vi "Deploy.vi"(8 "error in (no error)":errorcluster, 11 "SDIST in":refnum<class "NI_AB_API_DSDIST.lvclass">) -> (0 "error out":errorcluster, 3 "SDIST out":refnum<class "NI_AB_API_DSDIST.lvclass">)   [LabVIEW 2020, in "NI_AB_API_DSDIST.lvclass"]
uses:
  <vilib>/AppBuilder/AB_API/DSDIST/NI_AB_API_DSDIST.lvclass
  <vilib>/AppBuilder/AB_API/DSDIST/NI_AB_API_DSDIST.lvclass/NI_AB_API_DSDIST.ctl
  <vilib>/AppBuilder/AB_API/Build/NI_AB_API_Build.lvclass
  e:/builds/penguin/labview/branches/2020/dev/dist/vi.lib/AppBuilder/AB_API/SDIST/NI_AB_API_SDIST.lvclass
  e:/builds/penguin/labview/branches/2020/dev/dist/vi.lib/AppBuilder/AB_API/Build/NI_AB_API_Build.lvclass
  e:/builds/penguin/labview/branches/2020/dev/dist/vi.lib/AppBuilder/AB_API/DSDIST/NI_AB_API_DSDIST.lvclass
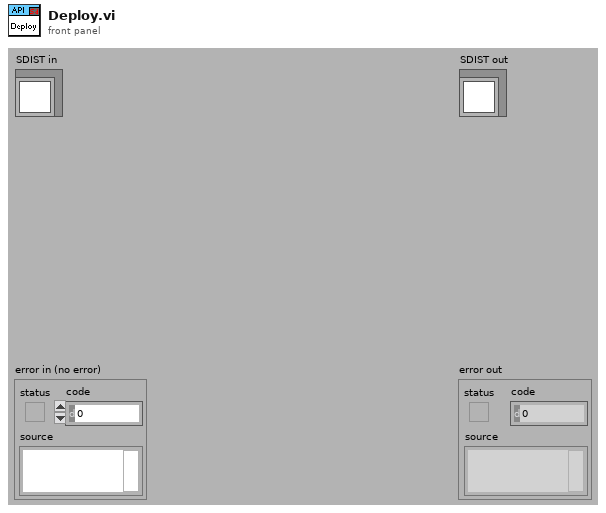
[diagram p1: front panel]
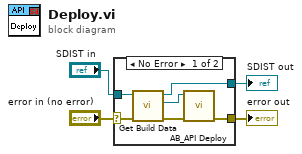
[diagram p0: block diagram]
diagram:
  n1 = case shown="No Error" "error in (no error)" {
    selector: "error in (no error)" -> [w6 w12]
    tunnel: [w10 w12] -> w3
    tunnel: [w8 w11] -> w1
    tunnel: "SDIST in" -> [w9 w11]
    frame No Error {
      n2 = call <vilib>:"Get Build Data.vi"("error in (no error)"=w6, "NI_AB_API_Build in"=w9) -> ("error out"=w5:errorcluster, "AB_Build.lvclass"=w7:refnum<class "AB_Build.lvclass">, "NI_AB_API_Build out"=w8:refnum<class "NI_AB_API_DSDIST.lvclass">)  [unwired: 7 in]
      n3 = call <vilib>:"AB_API Deploy.vi"("error in (no error)"=w5, "Build in"=w7) -> ("error out"=w10:errorcluster)  [unwired: 8 in, 1 out]
    }
    frame Error {
    }
  }
  "error out" <- w3
  "SDIST out" <- w1
